vi "Get CD Execution Mode type string.vi"(8 "error in (no error)":errorcluster, 11 "CD Execution Mode":T1) -> (0 "error out":errorcluster, 3 "Execution Mode type":string="Timing and Sync NewCD.xml")   [LabVIEW 2014, in "CD model script.lvlib"]
doc: "Get the execution mode type as string. You need the execution mode type to copy the build .LLB to the correct VeriStand folder.\n\n<B>Execution Mode - Execution Mode string</B>\nAsynchronous - <B>Custom Devices</B>\nInline HW Interface - <B>Custom Devices</B>\nInline Model Interface - <B>Custom Devices</B>\nInline Timing and Sync - <B>Timing and Sync</B>\nAsynchronous Timing and Sync - <B>Timing and Sync</B>"
uses:
  CD model script.lvlib
  CD Wizard - Execution Mode.ctl
  <vilib>/NI Veristand/Custom Device API/Custom Device Execution Mode.ctl
  Constants/Constants TypDef/Common.ctl
  Constants/Common.vi
  <vilib>/NI Veristand/Custom Device API/Custom Device API.lvlib
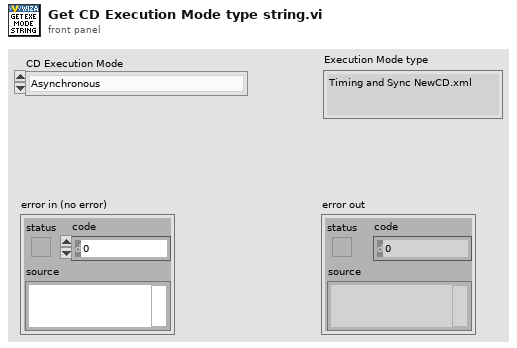
[diagram p1: front panel]
types:
  T1 = typedef "CD model script.lvlib/CD Wizard - Execution Mode.ctl" = enum16{"Asynchronous", "Inline HW Interface", "Inline Model Interface", "Inline Timing and Sync", "Asynchronous Timing and Sync"}
  T2 = typedef "CD model script.lvlib/Common.ctl" = enum16{"ProjectName", "TemplatesFolderName", "ProjectTemplatePathAndName", "ReadmeTemplatePathAndName", "TimingAndSyncFolderName", "CustomDeviceFolderName"}
  T3 = typedef "Custom Device API.lvlib/Custom Device Execution Mode.ctl" = enum16{"Asynchronous", "Inline HW Interface", "Inline Model Interface", "Inline Timing and Sync", "Asynchronous Timing and Sync"}
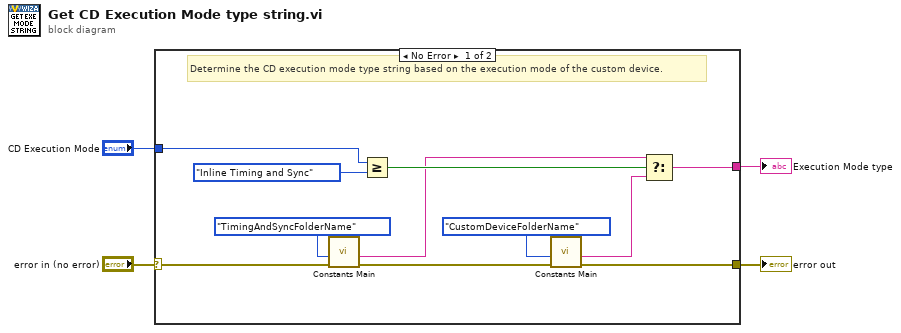
[diagram p0: block diagram]
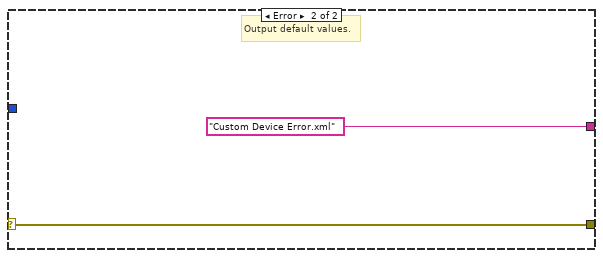
[diagram p2: hidden frame]
diagram:
  n1 = case shown="No Error" "error in (no error)" {
    selector: "error in (no error)" -> [w10 w17]
    tunnel: "CD Execution Mode" -> [w9 _]
    tunnel: [w8 w17] -> w2
    tunnel: [w7 "Custom Device Error.xml"] -> w1
    frame No Error {
      # "Determine the CD execution mode type string based on the execution mode of the custom device."
      n2 = call-poly "Constants Main.vi"("error in (no error)"=w10, "Action"=Common."TimingAndSyncFolderName") -> ("error out"=w13:errorcluster, "Output"=w12:string)  [unwired: 8 in]
      n3 = Greater Or Equal?(x=w9, y=Custom_Device_Execution_Mode."Inline Timing and Sync" ("CD Execution Mode")) -> (x >= y?=w14:bool)
      n4 = call-poly "Constants Main.vi"("error in (no error)"=w13, "Action"=Common."CustomDeviceFolderName") -> ("error out"=w8:errorcluster, "Output"=w11:string)  [unwired: 8 in]
      n5 = Select(t=w12, s=w14, f=w11) -> (s? t:f=w7:string)
    }
    frame Error {
      # "Output default values."
    }
  }
  "error out" <- w2
  "Execution Mode type" <- w1
